vi "HMI.vi"(8 "error in (no error)":errorcluster caption="entrée d'erreur (pas d'erreur)", 11 "Popup Operator_Input Batch In":refnum<class "Class Popup Operator_Input_PCRE.lvclass">) -> (0 "error out":errorcluster caption="sortie d'erreur", 1 "Input":string="Attente \nvalidation", 2 "Operator_Selection":bool, 3 "Popup Operator_Input Batch In":refnum<class "Class Popup Operator_Input_PCRE.lvclass">)   [LabVIEW 2020, in "Library Instrument & Equipement.lvlib" / "Library Popup.lvlib" / "Class Popup Operator_Input_PCRE.lvclass"]
uses:
  Class Popup Operator_Input_PCRE.lvclass
  C:/Users/ngarcin/OneDrive - Altyor/Standard TB/Class/Popup/Class Popup (Main)/Class Popup (Main).lvclass
  <vilib>/regexp/Match Regular Expression.xnode
  Class Popup (Main)/Class Popup (Main).lvclass
  Class Popup Operator_Input_PCRE.lvclass/Class Popup Operator_Input_PCRE.ctl
panel:
  in  "Bouton NOK":bool
  in  "Input OP":string="Attente \nvalidation"
  in  "Bouton OK":bool
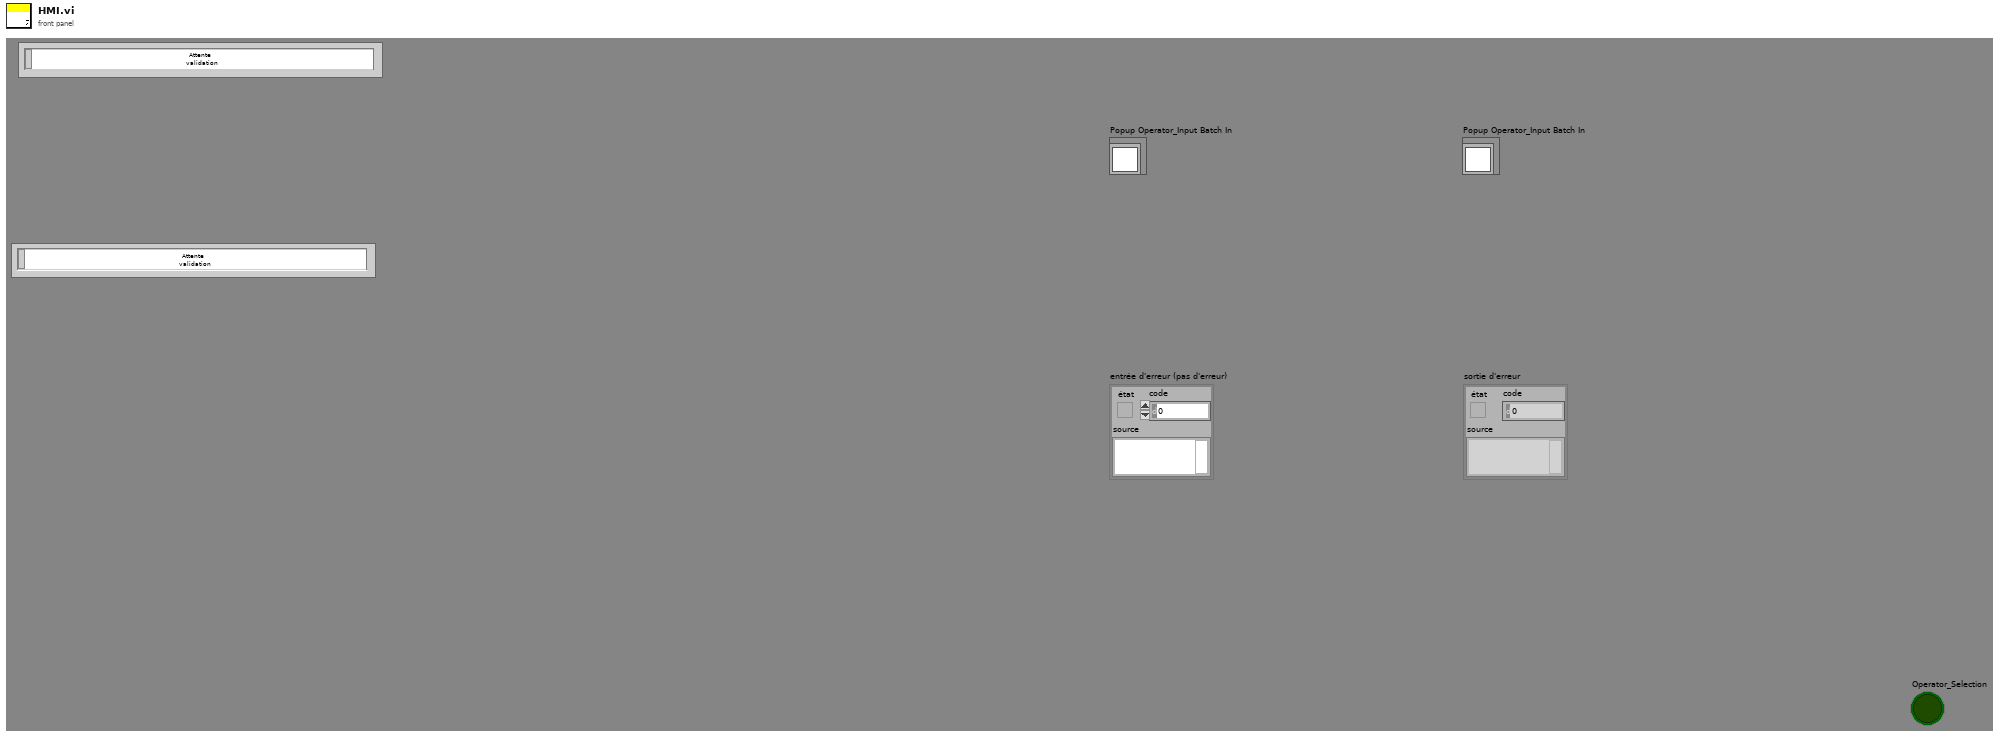
[diagram p1: front panel]
types:
  T1 = enum32{"Invalid", "Standard", "Closed", "Hidden", "Minimized", "Maximized"}
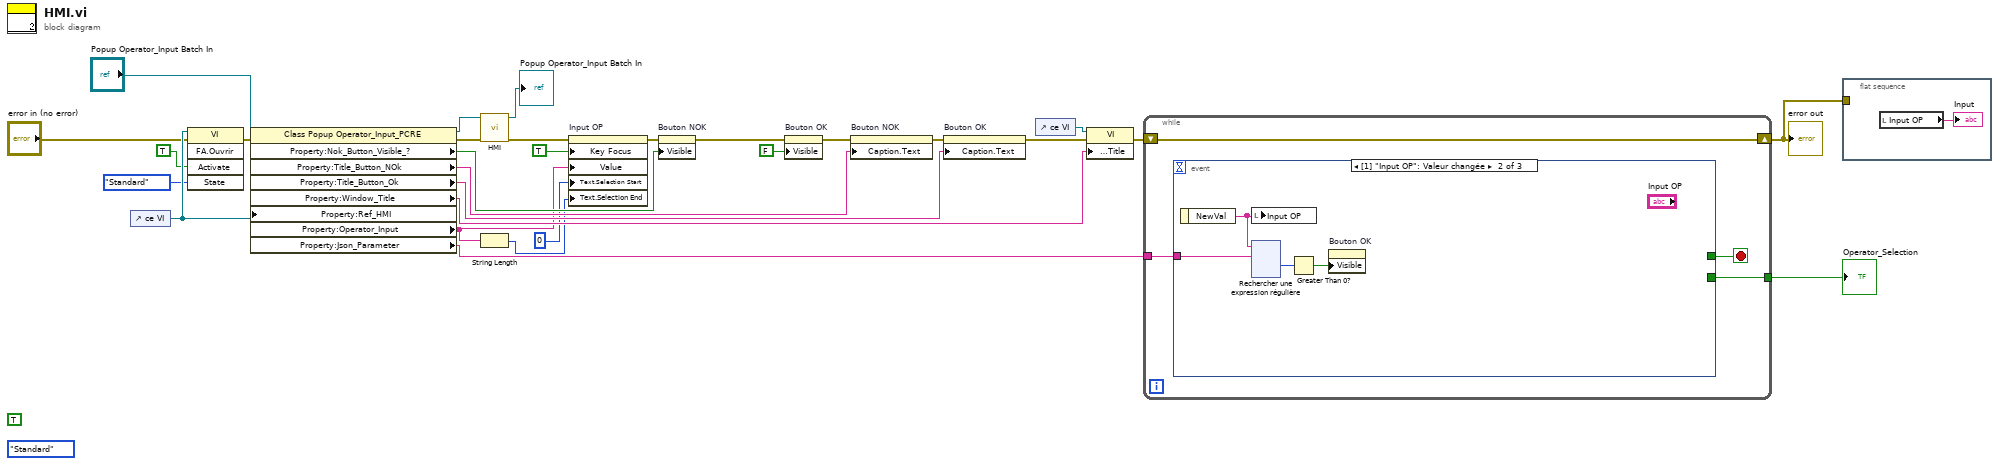
[diagram p0: block diagram]
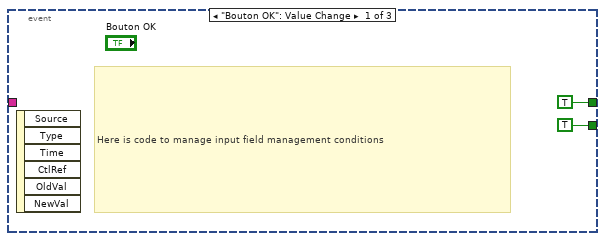
[diagram p2: hidden frame]
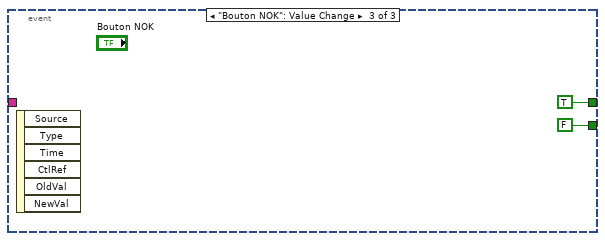
[diagram p3: hidden frame]
diagram:
  (unwired) T1."Standard" ("État")
  (unwired) TRUE ("Activer ?")
  n1 = control-ref of="ce VI"() -> (w9:refnum<vi>)
  n2 = invoke class="VI" method="FA.Ouvrir"(reference=w9, error in="error in (no error)", "Activate"=TRUE ("Activer ?"), "State"=T1."Standard" ("État")) -> (error out=w6:errorcluster)  [unwired: 1 in, 4 out]
  n3 = property class="Class Popup Operator_Input_PCRE"(reference="Popup Operator_Input Batch In", error in=w6, "Property:Ref_HMI"=w9) -> (reference out=w24:refnum<class "Class Popup Operator_Input_PCRE.lvclass">, error out=w4:errorcluster, "Property:Nok_Button_Visible_?"=w29:bool, "Property:Title_Button_NOk"=w23:string, "Property:Title_Button_Ok"=w21:string, "Property:Window_Title"=w26:string, "Property:Operator_Input"=w13:string, "Property:Json_Parameter"=w1:string)
  n4 = call-parent "HMI.vi"("error in (no error)"=w4, "Class Popup (Main) en entrée"=w24) -> ("error out"=w3:errorcluster, "Class Popup (Main) en sortie"=→"Popup Operator_Input Batch In":refnum<class "Class Popup Operator_Input_PCRE.lvclass">)  [unwired: 6 in, 2 out]
  n5 = String Length(string=w13) -> (length=w15:i32)
  n6 = property on="Input OP" class="Ch"(error in=w3, "Key Focus"=TRUE ("Focus clavier"), "Value"=w13, "Text.Selection Start"=u32 0 ("Texte.Sélection:Début"), "Text.Selection End"=w15) -> (error out=w2:errorcluster)  [unwired: 1 in, 1 out]
  n7 = property on="Bouton NOK" class="Bool"(error in=w2, "Visible"=w29) -> (error out=w19:errorcluster)  [unwired: 1 in, 1 out]
  n8 = property on="Bouton OK" class="Bool"(error in=w19, "Visible"=FALSE ("Activer ?")) -> (error out=w18:errorcluster)  [unwired: 1 in, 1 out]
  n9 = property on="Bouton NOK" class="Bool"(error in=w18, "Caption.Text"=w23) -> (error out=w22:errorcluster)  [unwired: 1 in, 1 out]
  n10 = property on="Bouton OK" class="Bool"(error in=w22, "Caption.Text"=w21) -> (error out=w16:errorcluster)  [unwired: 1 in, 1 out]
  n11 = control-ref of="ce VI"() -> (w27:refnum<vi>)
  n12 = property class="VI"(reference=w27, error in=w16, "Front Panel.Title"=w26) -> (error out=w25:errorcluster)  [unwired: 1 out]
  n13 = while {
    tunnel: [w31] -> w28
    shift-right: [w32] -> w12
    shift-left: w25 -> [w32]
    tunnel: w1 -> [w30]
    stop <- w33 stop-if-true
    n14 = event shown="[1] \"Input OP\": Valeur changée" {
      selector: _ -> [_ _ _]
      dyn-events: _ -> [_ _ _]
      timeout: _ -> [_ _ _]
      tunnel: [TRUE ("Valeur (Signalisation)") _ TRUE ("Valeur (Signalisation)")] -> w33
      tunnel: [TRUE ("Operator_Selection") _ FALSE ("Operator_Selection")] -> w31
      tunnel: w30 -> [_ w38 _]
      event "Bouton OK": Value Change {
        # "Here is code to manage input field management conditions"
        n15 = event-data() -> ()  [unwired: 1 in, 6 out]
      }
      event "Input OP": Value Change {
        n16 = event-data() -> ("NewVal"=w39:string)  [unwired: 1 in]
        n17 = local write "Input OP"(w39) -> ()
        n18 = xnode "Rechercher une expression régulière"("chaîne en entrée"=w39, "expression régulière"=w38) -> ("offset après correspondance"=w37:i32)  [unwired: 4 in, 4 out]
        n19 = Greater Than 0?(x=w37) -> (x > 0?=w36:bool)
        n20 = property on="Bouton OK" class="Bool"("Visible"=w36) -> ()  [unwired: 2 in, 2 out]
      }
      event "Bouton NOK": Value Change {
        n21 = event-data() -> ()  [unwired: 1 in, 6 out]
      }
    }
  }
  "error out" <- w12
  "Operator_Selection" <- w28
  n22 = flat-sequence {
    tunnel: w12 -> [_]
    frame #0 {
      n23 = local read "Input OP"() -> (→"Input":string)
    }
  }
